vi "Get ViName.vi"(8 "error in":errorcluster caption="错误输入（无错误）", 11 "VI*":refnum<vi>) -> (0 "error out":errorcluster caption="错误输出", 2 "VI Name":string, 3 "VI* out":refnum<vi>)   [LabVIEW 2013, in "PanelDataNode.lvclass"]
uses:
  PanelDataNode.lvclass
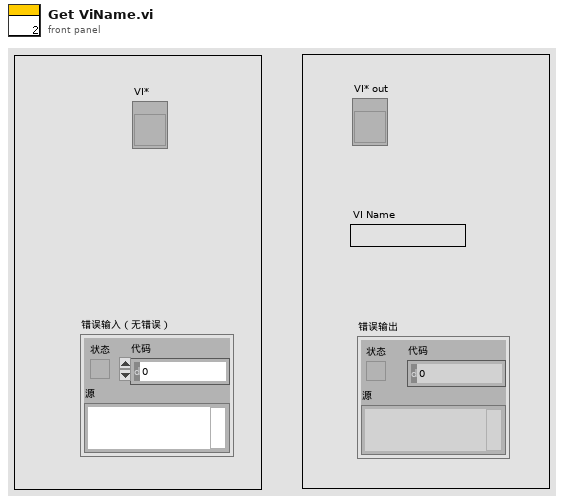
[diagram p1: front panel]
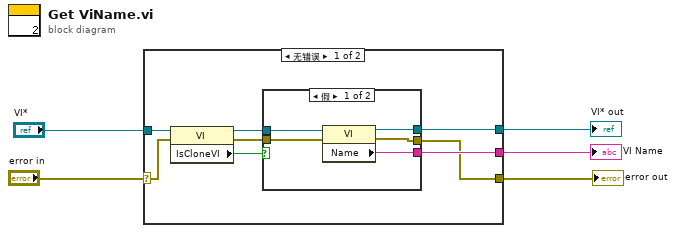
[diagram p0: block diagram]
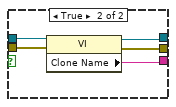
[diagram p2: hidden frame]
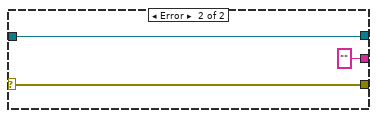
[diagram p3: hidden frame]
diagram:
  n1 = case shown="无错误" "error in" {
    selector: "error in" -> [w8 w26]
    tunnel: "VI*" -> [w13 w25]
    tunnel: [w10 "" ("Clone Name")] -> w4
    tunnel: [w9 w25] -> w3
    tunnel: [w6 w26] -> w1
    frame No Error {
      n2 = property class="VI"(reference=w13, error in=w8) -> (reference out=w11:refnum<vi>, error out=w7:errorcluster, "IsCloneVI"=w12:bool)
      n3 = case shown="假" w12 {
        tunnel: w11 -> [w18 w23]
        tunnel: [w17 w21] -> w10
        tunnel: [w16 w22] -> w9
        tunnel: w7 -> [w15 w20]
        tunnel: [w14 w19] -> w6
        frame False {
          n4 = property class="VI"(reference=w18, error in=w15) -> (reference out=w16:refnum<vi>, error out=w14:errorcluster, "Name"=w17:string)
        }
        frame True {
          n5 = property class="VI"(reference=w23, error in=w20) -> (reference out=w22:refnum<vi>, error out=w19:errorcluster, "Clone Name"=w21:string)
        }
      }
    }
    frame Error {
    }
  }
  "VI Name" <- w4
  "VI* out" <- w3
  "error out" <- w1
